vi "tcp_load_cal_file.vi"(0 "connection_id_in":refnum<k5>, 1 "button_tcp_load_cal":bool, 5 "sva_ready":bool, 7 "cal_file":string, 9 "tcp_connected_in":bool, 11 "error in":errorcluster) -> (4 "connection_id_out":refnum<k5>, 10 "tcp_connected_out":bool, 15 "error out":errorcluster)   [LabVIEW 2025]
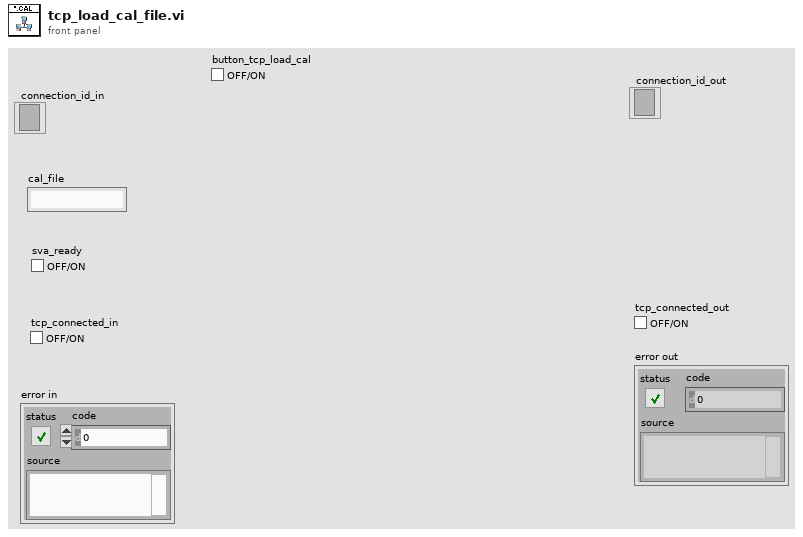
[diagram p1: front panel]
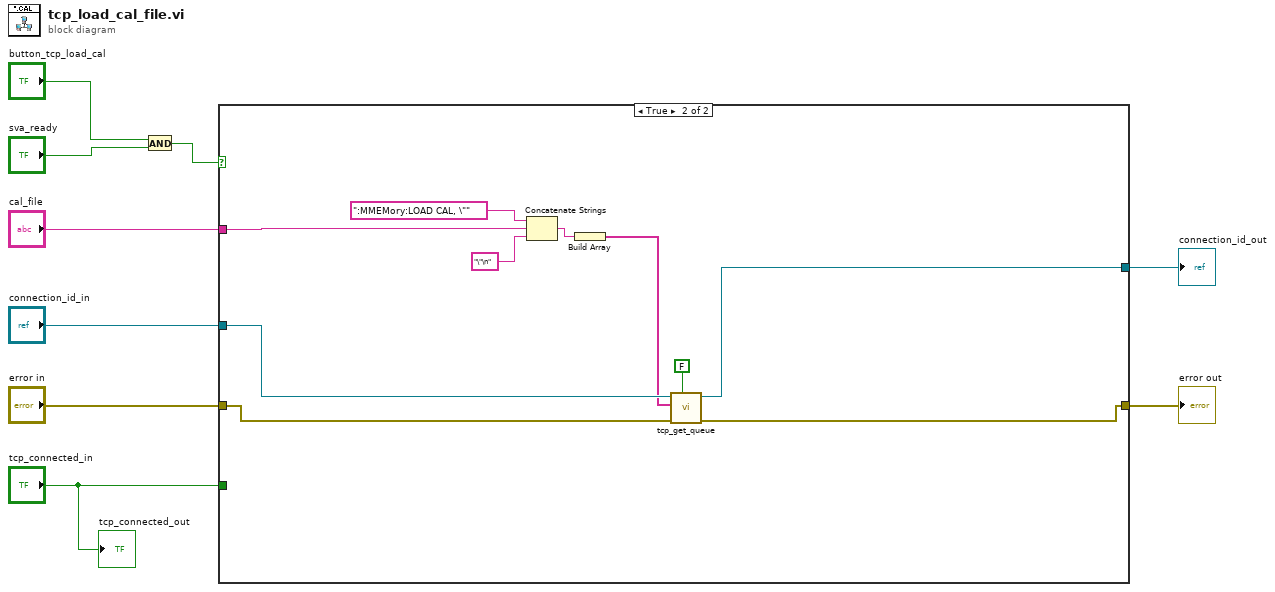
[diagram p0: block diagram]
diagram:
  n1 = And(x="button_tcp_load_cal", y="sva_ready") -> (x .and. y?=w9:bool)
  n2 = case shown="True" w9 {
    tunnel: [w10 w12] -> w7
    tunnel: [w11 w21] -> w6
    tunnel: "connection_id_in" -> [w11 w20]
    tunnel: "error in" -> [w10 w19]
    tunnel: "tcp_connected_in" -> [_ _]
    tunnel: "cal_file" -> [_ w14]
    frame False {
    }
    frame True {
      n3 = Concatenate Strings(":MMEMory:LOAD CAL, \"", w14, "\"\n" ("string")) -> (w16:string)
      n4 = Build Array(w16) -> (w15:string[])
      n5 = call "tcp_get_queue.vi"("response?"=FALSE, "error in"=w19, "command queue"=w15, "connection in"=w20) -> ("error out"=w12:errorcluster, "connection out"=w21:refnum<k5>)  [unwired: 5 in, 1 out]
    }
  }
  "error out" <- w7
  "connection_id_out" <- w6
  "tcp_connected_out" <- "tcp_connected_in"
